vi "ExTestReadingF32FromImageExample.vi"() -> ()   [LabVIEW 2010]
panel:
  out "Test 2d Array":sgl[][](array[numeric]) format="%.2f"
  out "Test 1d array":sgl[](array[numeric]) format="%.2f"
  out "Pixel Value u16":u16
  out "Pixel Value i32":i32
  out "Pixel Value f32":sgl format="%.2f"
  out "error out":errorcluster
  in  "error in (no error)":errorcluster
  # "ExTestReadingFromImageExample\nThis example shows how to pull the data out of the\nToolkit data handle into the LabView world.\nThis specific example shows it for 32 bit float.\nAfter running this example the right allows you to \nlook at ramp that was created."
  # "NOTICE\n\nTHIS VI REQUIRES THAT THE TOOLKIT\nBE UNLOADED BY RUNNING THE\n VI EXCLOSEGLOBALCAM.VI\n BEFORE LEAVING LABVIEW."
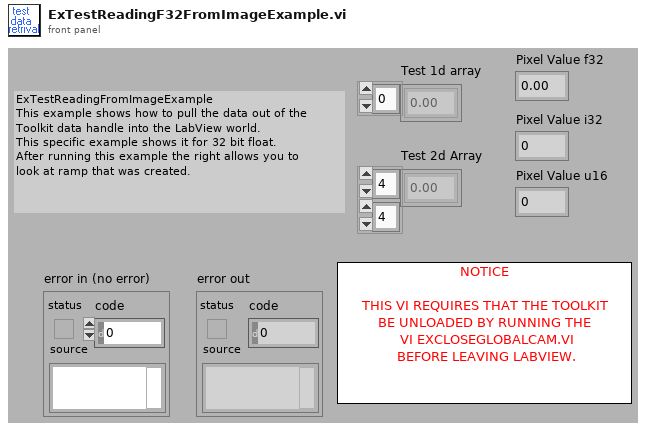
[diagram p1: front panel]
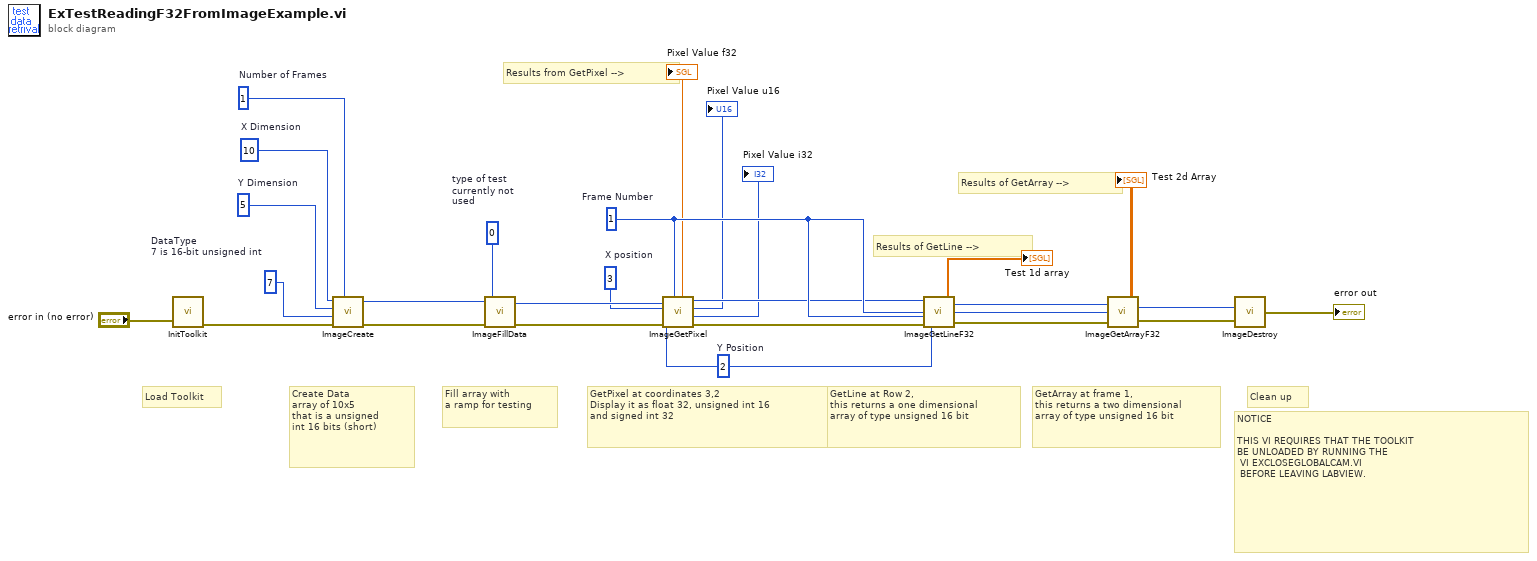
[diagram p0: block diagram]
diagram:
  w9 = 1  # Frame Number
  w12 = 2  # Y Position
  w13 = 3  # X position
  w15 = 0  # type of test currently not used
  w17 = 1  # Number of Frames
  w18 = 10  # X Dimension
  w19 = 5  # Y Dimension
  w20 = 7  # DataType  7 is 16-bit unsigned int
  # "NOTICE\n\nTHIS VI REQUIRES THAT THE TOOLKIT\nBE UNLOADED BY RUNNING THE\n VI EXCLOSEGLOBALCAM.VI\n BEFORE LEAVING LABVIEW."
  # "Clean up"
  # "Results of GetArray -->"
  # "GetArray at frame 1,\nthis returns a two dimensional\narray of type unsigned 16 bit"
  # "GetLine at Row 2,\nthis returns a one dimensional\narray of type unsigned 16 bit"
  # "Results of GetLine -->"
  # "GetPixel at coordinates 3,2\nDisplay it as float 32, unsigned int 16\nand signed int 32"
  # "Results from GetPixel -->"
  # "Fill array with \na ramp for testing"
  # "Create Data\narray of 10x5\nthat is a unsigned \nint 16 bits (short)"
  # "Load Toolkit"
  n1 = call <userlib>:"InitToolkit.vi"("error in"="error in (no error)") -> ("error out"=w26:errorcluster)
  n2 = call <userlib>:"ImageCreate.vi"("X dimension"=w18, "Y dimension"=w19, "Data Type"=w20, "error in"=w26, "Number Of Frames"=w17) -> ("Image Handle"=w16:u32, "error out"=w24:errorcluster)
  n3 = call <userlib>:"ImageFillData.vi"("error in"=w24, "Type of Test"=w15, "Image Handle"=w16) -> ("error out"=w23:errorcluster, "Image Handle"=w14:u32)
  n4 = call <userlib>:"ImageGetPixel.vi"("Z position"=w9, "error in"=w23, "Y position"=w12, "X position"=w13, "Data Handle"=w14) -> ("error out"=w7:errorcluster, "Pixel Value i32"=→"Pixel Value i32":i32, "Pixel Value u16"=→"Pixel Value u16":u16, "Data Handle"=w8:u32, "Pixel Value f32"=→"Pixel Value f32":sgl)
  n5 = call <userlib>:"ImageGetLineF32.vi"("error in"=w7, "Z Position"=w9, "Y Position"=w12, "Data Handle"=w8) -> ("error out"=w22:errorcluster, "Array F32"=→"Test 1d array":sgl[], "Data Handle"=w11:u32)
  n6 = call <userlib>:"ImageGetArrayF32.vi"("error in"=w22, "Z position"=w9, "Image Handle"=w11) -> ("error out"=w21:errorcluster, "Array Float 32"=→"Test 2d Array":sgl[][], "Image Handle"=w10:u32)
  n7 = call <userlib>:"ImageDestroy.vi"("error in"=w21, "Data handle"=w10) -> ("error out"=→"error out":errorcluster)
